vi "Configure Channel (Math).vi"(0 "VISA resource name":refnum<visa-resource-name>, 1 "Computing Equation (\"0001\")":string="0001", 5 "Math Channel (001)":string="001", 7 "Enable Channel (False)":bool, 9 "Span":T1={"Enable Span (False)"=FALSE, "Decimal Place (2)"=2, "Lower Span (0.00)"=0.0, "Upper Span (100.00)"=100.0, "Unit Character (\"\")"=""} {"Upper Span (100.00)" min=-9999999.0 max=99999999.0 format="%#_8g"; "Lower Span (0.00)" min=-9999999.0 max=99999999.0 format="%#_8g"; "Decimal Place (2)" min=0 max=5 step=1}, 11 "error in (no error)":errorcluster) -> (4 "VISA resource name out":refnum<visa-resource-name>, 6 "Math Channel":string, 15 "error out":errorcluster)   [LabVIEW 2020, in "Yokogawa GX Series.lvlib"]
doc: "Sets the computing equation.\n\nCommand: SRangeMath"
uses:
  <instrlib>/Yokogawa GX Series/Yokogawa GX Series.lvlib
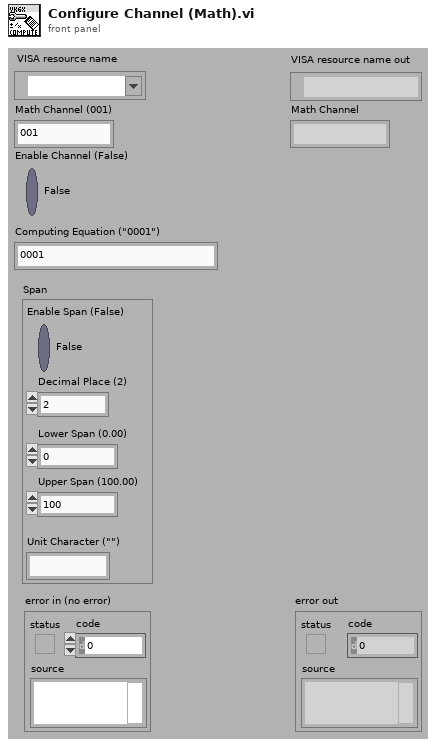
[diagram p1: front panel]
types:
  T1 = cluster{"Enable Span (False)":bool, "Decimal Place (2)":i32, "Lower Span (0.00)":dbl, "Upper Span (100.00)":dbl, "Unit Character (\"\")":string}
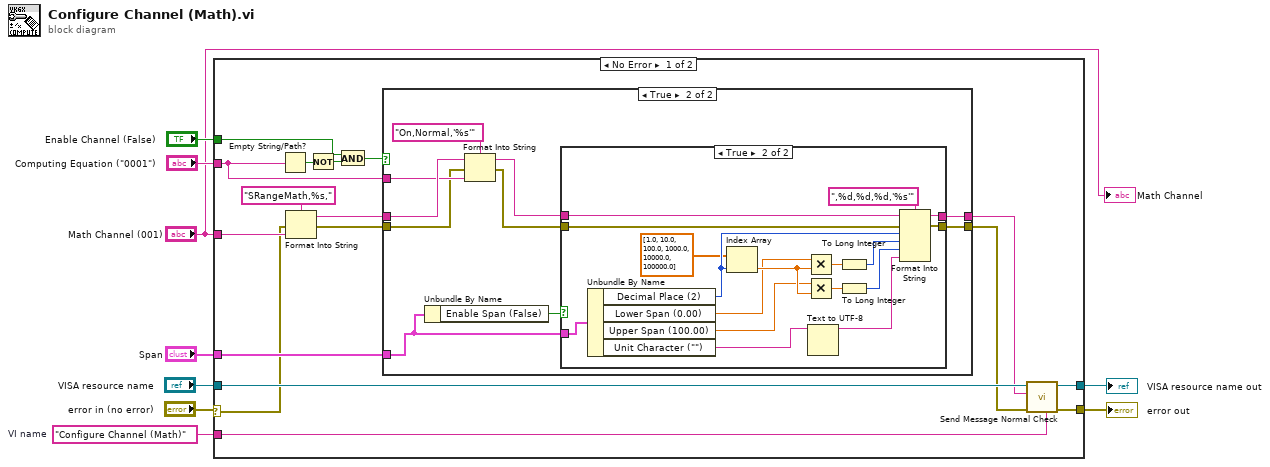
[diagram p0: block diagram]
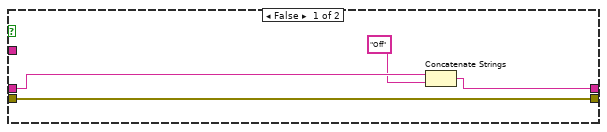
[diagram p2: hidden frame]
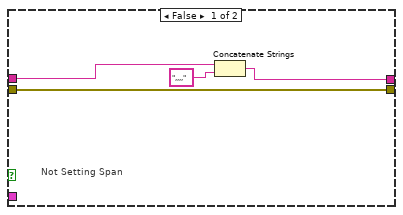
[diagram p3: hidden frame]
diagram:
  w4 = "Configure Channel (Math)"  # VI name
  n1 = case shown="No Error" "error in (no error)" {
    selector: "error in (no error)" -> [w10 w62]
    tunnel: "Computing Equation (\"0001\")" -> [w24 _]
    tunnel: "Enable Channel (False)" -> [w23 _]
    tunnel: "Span" -> [w20 _]
    tunnel: [w19 w63] -> w6
    tunnel: "VISA resource name" -> [w18 w63]
    tunnel: w4 -> [w15 _]
    tunnel: "Math Channel (001)" -> [w12 _]
    tunnel: [w11 w62] -> w2
    frame No Error {
      n2 = Empty String/Path?(string/path=w24) -> (empty?=w21:bool)
      n3 = Format Into String(format string="SRangeMath,%s,", error in=w10, w12) -> (resulting string=w13:string, error out=w25:errorcluster)  [unwired: 1 in]
      n4 = Not(x=w21) -> (.not. x?=w22:bool)
      n5 = And(x=w23, y=w22) -> (x .and. y?=w14:bool)
      n6 = case shown="True" w14 {
        tunnel: w25 -> [w27 w33]
        tunnel: w24 -> [_ w34]
        tunnel: w20 -> [_ w38]
        tunnel: [w27 w40] -> w17
        tunnel: [w28 w39] -> w16
        tunnel: w13 -> [w30 w36]
        frame False {
          n7 = Concatenate Strings(w30, "Off") -> (w28:string)
        }
        frame True {
          n8 = Unbundle By Name(w38) -> ("Enable Span (False)"=w37:bool)
          n9 = Format Into String(format string="On,Normal,'%s'", initial string=w36, error in=w33, w34) -> (resulting string=w31:string, error out=w32:errorcluster)
          n10 = case shown="True" w37 {
            tunnel: w32 -> [w44 w60]
            tunnel: [w44 w59] -> w40
            tunnel: w31 -> [w43 w48]
            tunnel: [w41 w58] -> w39
            tunnel: w38 -> [_ w54]
            frame False {
              # "Not Setting Span"
              n11 = Concatenate Strings(w43, ",,,,") -> (w41:string)
            }
            frame True {
              n12 = Unbundle By Name(w54) -> ("Decimal Place (2)"=w51:i32, "Lower Span (0.00)"=w53:dbl, "Upper Span (100.00)"=w52:dbl, "Unit Character (\"\")"=w46:string)
              n13 = Index Array(array=dbl[] [1.0, 10.0, 100.0, 1000.0, 10000.0, 100000.0], index=w51) -> (element=w57:dbl)
              n14 = Multiply(x=w53, y=w57) -> (x*y=w56:dbl)
              n15 = Multiply(x=w52, y=w57) -> (x*y=w55:dbl)
              n16 = Text to UTF-8(11:w46) -> (3:w45:string)  [unwired: 2 in, 1 out]
              n17 = To Long Integer(number=w56) -> (32bit integer=w50:i32)
              n18 = To Long Integer(number=w55) -> (32bit integer=w49:i32)
              n19 = Format Into String(format string=",%d,%d,%d,'%s'", initial string=w48, error in=w60, w51, w50, w49, w45) -> (resulting string=w58:string, error out=w59:errorcluster)
            }
          }
        }
      }
      n20 = call <instrlib>:"Send Message Normal Check.vi"("Source (\"\")"=w15, "error in (no error)"=w17, "Send Message (\"\")"=w16, "VISA resource name"=w18) -> ("error out"=w11:errorcluster, "VISA resource name out"=w19:refnum<visa-resource-name>)  [unwired: 2 in, 4 out]
    }
    frame Error {
    }
  }
  "error out" <- w2
  "VISA resource name out" <- w6
  "Math Channel" <- "Math Channel (001)"
